vi "Start.vi"(8 "Error In":errorcluster, 11 "reference in":refnum<class "Camera.lvclass">) -> (0 "Error Out":errorcluster, 3 "reference out":refnum<class "Camera.lvclass">)   [LabVIEW 2025, in "Camera.lvclass"]
uses:
  Camera.lvclass
  Camera Worker/Camera Worker.lvclass
  Interfaces/IRead Image/IRead Images/IRead Image.lvclass
  Camera Worker/Camera Worker.lvclass/Camera Worker.ctl
  Interfaces/IRunnable/IRunnable.lvclass
  Interfaces/IConfigure/IConfigure.lvclass
  Interfaces/IConfiguration/IConfiguration.lvclass
  <vilib>/ActorFramework/Actor/Actor.lvclass
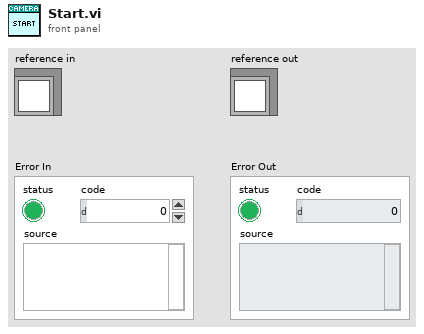
[diagram p1: front panel]
types:
  T1 = typedef "Camera.lvclass/ObjectAttributes.ctl" = cluster{"IConfigure":refnum<class "IConfigure.lvclass">, "Worker Enqueuer":refnum<class "Message Enqueuer.lvclass">, "Start Counter":i32, "Initialized":bool}
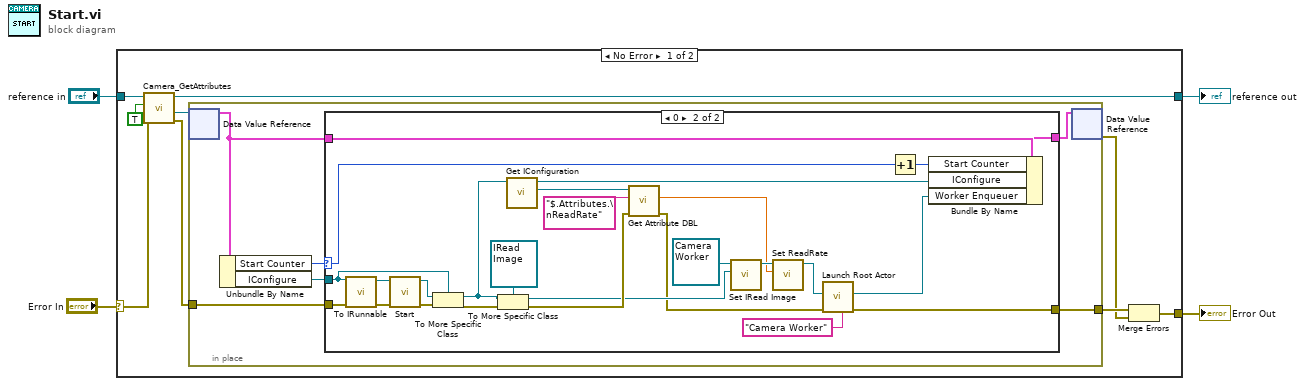
[diagram p0: block diagram]
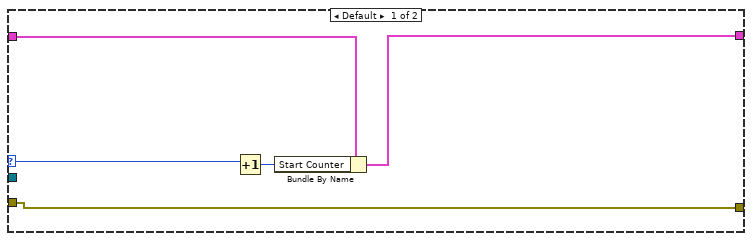
[diagram p2: hidden frame]
diagram:
  n1 = case shown="No Error" "Error In" {
    selector: "Error In" -> [w13 w52]
    tunnel: [w5 w52] -> w3
    tunnel: [w11 w51] -> w1
    tunnel: "reference in" -> [w12 w51]
    frame No Error {
      n2 = call "Camera_GetAttributes.vi"("Error In"=w13, "OnlyGetDvrReference(False)"=TRUE, "reference in"=w12) -> ("Error Out"=w8:errorcluster, "DataRef"=w9:refnum<data-value>, "reference out"=w11:refnum<class "Camera.lvclass">)  [unwired: 5 in, 1 out]
      n3 = in-place {
        in-place-border: w8 -> [w17]
        in-place-border: [w14] -> w7
        n4 = in-place-dvr #1(w9) -> (w16:T1)  [unwired: 1 out]
        n5 = Unbundle By Name(w16) -> ("Start Counter"=w19:i32, "IConfigure"=w18:refnum<class "IConfigure.lvclass">)
        n6 = case shown="0" w19 {
          selector: w19 -> [w23 w30]
          tunnel: w18 -> [_ w45]
          tunnel: w17 -> [w20 w50]
          tunnel: w16 -> [w22 w32]
          tunnel: [w21 w31] -> w15
          tunnel: [w20 w26] -> w14
          frame Default {
            n7 = Increment(x=w23) -> (x+1=w24:i32)
            n8 = Bundle By Name(cluster=w22, "Start Counter"=w24) -> (w21:T1)
          }
          frame 0 {
            n9 = call "To IRunnable.vi"("error in"=w50, "LabVIEW Object"=w45) -> ("error out"=w49:errorcluster, "IRunnable"=w48:refnum<class "IRunnable.lvclass">)  [unwired: 8 in]
            n10 = call-dynamic "Start.vi"("error in"=w49, "IRunnable in"=w48) -> ("error out"=w47:errorcluster, "IRunnable out"=w46:refnum<class "IRunnable.lvclass">)  [unwired: 8 in]
            n11 = To More Specific Class(target class=w45, reference=w46, error in=w47) -> (specific class reference=w38:refnum<class "IConfigure.lvclass">, error out=w39:errorcluster)
            n12 = To More Specific Class(target class=refnum<class "IRead Image.lvclass"> refnum ("IRead Image.lvclass"), reference=w38, error in=w39) -> (specific class reference=w37:refnum<class "IRead Image.lvclass">, error out=w40:errorcluster)
            n13 = call-dynamic "Get IConfiguration.vi"("IConfigure in"=w38) -> ("IConfiguration"=w42:refnum<class "IConfiguration.lvclass">, "IConfigure out"=w28:refnum<class "IConfigure.lvclass">)  [unwired: 9 in]
            n14 = call-dynamic "Get Attribute DBL.vi"("error in"=w40, "Attribute"="$.Attributes.\nReadRate", "IConfiguration in"=w42) -> ("error out"=w33:errorcluster, "Value"=w35:dbl)  [unwired: 6 in, 1 out]
            n15 = call "Set IRead Image.vi"("IRead Image"=w37, "Worker in"=refnum<class "Camera Worker.lvclass"> refnum ("Camera Worker.lvlib:Camera Worker.lvclass")) -> ("Worker out"=w36:refnum<class "Camera Worker.lvclass">)  [unwired: 9 in]
            n16 = call "Set ReadRate.vi"("ReadRate"=w35, "Worker in"=w36) -> ("Worker out"=w34:refnum<class "Camera Worker.lvclass">)  [unwired: 9 in]
            n17 = call <vilib>:"Launch Root Actor.vi"("Debug Alias"="Camera Worker", "error in (no error)"=w33, "Actor"=w34) -> ("error out"=w26:errorcluster, "Actor's Enqueuer"=w27:refnum<class "Message Enqueuer.lvclass">)  [unwired: 7 in]
            n18 = Increment(x=w30) -> (x+1=w29:i32)
            n19 = Bundle By Name(cluster=w32, "Start Counter"=w29, "IConfigure"=w28, "Worker Enqueuer"=w27) -> (w31:T1)
          }
        }
        n20 = in-place-dvr #1(w15) -> (w6:errorcluster)  [unwired: 1 out]
      }
      n21 = Merge Errors(w7, w6) -> (w5:errorcluster)
    }
    frame Error {
    }
  }
  "Error Out" <- w3
  "reference out" <- w1
